vi "TEST_DestinationFolder.vi"() -> ()   [LabVIEW 2020]
uses:
  ProligentResultProcessor/Datawarehouse/SetDestinationFolder.vi
  ProligentResultProcessor/Datawarehouse/Datawarehouse.lvclass
panel:
  out "error out":errorcluster
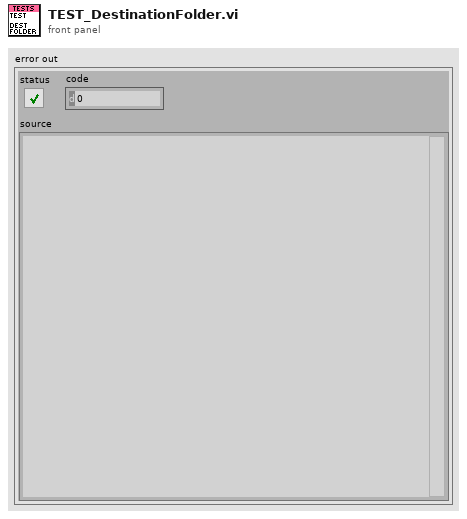
[diagram p1: front panel]
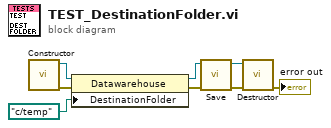
[diagram p0: block diagram]
diagram:
  n1 = call "Constructor.vi"() -> ("error out"=w7:errorcluster, "Datawarehouse"=w8:refnum<class "Datawarehouse.lvclass">)  [unwired: 10 in]
  n2 = property class="Datawarehouse"(reference=w8, error in=w7, "DestinationFolder"=path "c:/temp") -> (reference out=w4:refnum<class "Datawarehouse.lvclass">, error out=w6:errorcluster)
  n3 = call "Save.vi"("error in"=w6, "Datawarehouse in"=w4) -> ("error out"=w5:errorcluster, "Datawarehouse out"=w3:refnum<class "Datawarehouse.lvclass">)  [unwired: 8 in]
  n4 = call "Destructor.vi"("error in"=w5, "Datawarehouse"=w3) -> ("error out"=→"error out":errorcluster)  [unwired: 9 in]
